vi "Default Ini Config File.vi"() -> (3 "appended path":path)   [LabVIEW 2017, in "INI-Static-Variable-Support.lvlib"]
uses:
  INI-Static-Variable-Support.lvlib
  <userlib>/_NEVSTOP/Communicable State Machine(CSM)/addons/Logger/CSM File Logger.lvlib
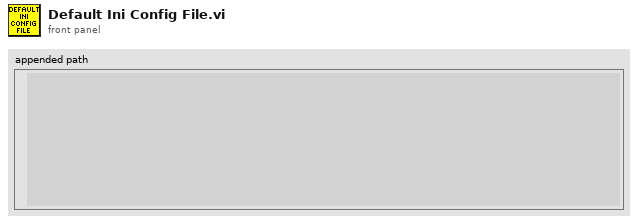
[diagram p1: front panel]
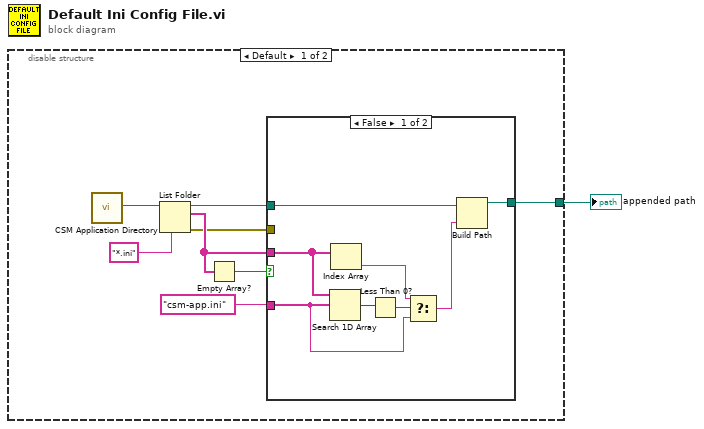
[diagram p0: block diagram]
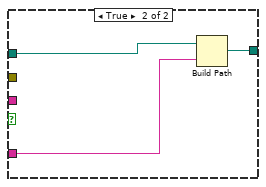
[diagram p2: hidden frame]
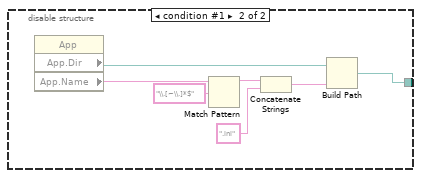
[diagram p3: hidden frame]
diagram:
  n1 = disable-structure shown="Default" {
    disable-tunnel: [w2 w21] -> w1
    frame condition #0 (active) {
      n2 = call <userlib>:"CSM Application Directory.vi"() -> ("CSM Application Dir"=w5:path)  [unwired: 11 in]
      n3 = List Folder(path=w5, pattern="*.ini") -> (path out=w8:path, filenames=w9:string[], error out=w6:errorcluster)  [unwired: 2 in, 1 out]
      n4 = Empty Array?(array=w9) -> (empty?=w7:bool)
      n5 = case shown="False" w7 {
        tunnel: w9 -> [w15 _]
        tunnel: w8 -> [w17 w20]
        tunnel: [w16 w19] -> w2
        tunnel: w6 -> [_ _]
        tunnel: "csm-app.ini" ("name or relative path") -> [w11 w18]
        frame False {
          n6 = Search 1D Array(1D array=w15, element=w11) -> (index of element=w14:i32)  [unwired: 1 in]
          n7 = Index Array(array=w15) -> (element=w12:string)  [unwired: 1 in]
          n8 = Less Than 0?(x=w14) -> (x < 0?=w13:bool)
          n9 = Select(t=w12, s=w13, f=w11) -> (s? t:f=w10:string)
          n10 = Build Path(base path=w17, name or relative path=w10) -> (appended path=w16:path)
        }
        frame True {
          n11 = Build Path(base path=w20, name or relative path=w18) -> (appended path=w19:path)
        }
      }
    }
    frame condition #1 {
      n12 = property class="App"() -> ("App.Dir"=w22:path, "App.Name"=w26:string)  [unwired: 2 in, 2 out]
      n13 = Match Pattern(string=w26, regular expression="\\.[~\\.]*$") -> (before substring=w27:string)  [unwired: 1 in, 3 out]
      n14 = Concatenate Strings(w27, ".ini" ("new ending (none)")) -> (w23:string)
      n15 = Build Path(base path=w22, name or relative path=w23) -> (appended path=w21:path)
    }
  }
  "appended path" <- w1
